vi "Logout.vi"(0 "User Manager Model in":refnum<class "User Manager Model.lvclass">, 11 "error in (no error)":errorcluster) -> (4 "User Manager Model out":refnum<class "User Manager Model.lvclass">, 15 "error out":errorcluster)   [LabVIEW 2017, in "User Manager Model.lvlib" / "User Manager Model.lvclass"]
uses:
  User Manager Model.lvclass
  C:/Program Files/National Instruments/LabVIEW 2017/vi.lib/gpm_packages/@cs/mva-core/Source/IModel/IModel/IModel.lvclass
  User Manager Model.lvclass/User Manager Model.ctl
  <vilib>/gpm_packages/@cs/persistence/source/XML/XML.lvclass
  C:/Program Files/National Instruments/LabVIEW 2017/vi.lib/gpm_packages/@cs/persistence/source/IPersist/IPersist.lvclass
  <vilib>/gpm_packages/@cs/user-manager/Source/iUser Configuration Manager/iUser Configuration Manager.lvclass
  <vilib>/gpm_packages/@cs/mva-core/Source/IObserver/IObserver/IObserver.lvclass/IObserver.ctl
  <vilib>/gpm_packages/@cs/mva-core/Source/IModel/IModel/IModel.lvclass/IModel.ctl
  <vilib>/gpm_packages/@cs/mva-core/Source/IMediator/PublishRequest/PublishRequest.lvclass/PublishRequest.ctl
  <vilib>/gpm_packages/@cs/mva-core/Source/IMediator/IMediator Messages/Publish Msg/Publish Msg.lvclass/Publish Msg.ctl
  <vilib>/gpm_packages/@cs/actor-framework-messages/Source/RoundTripMessage/RoundTripMessage.lvclass/RoundTripMessage.ctl
  <vilib>/ActorFramework/Message Enqueuer/Message Enqueuer.lvclass/Message Enqueuer.ctl
  <vilib>/gpm_packages/@cs/mva-core/Source/IMediator/IMediator Messages/Publish Msg/Send Pre-Addressed Publish.vi
  <vilib>/gpm_packages/@cs/mva-core/Source/IObserver/IObserver/Read Unique ID.vi
  <vilib>/gpm_packages/@cs/mva-core/Source/IMediator/PublishRequest/Pack Publish Request.vi
  <vilib>/gpm_packages/@cs/actor-framework-messages/Source/RoundTripMessage/Return Round-Trip Message.vi
  <vilib>/ActorFramework/Message Enqueuer/Enqueue.vi
  <vilib>/gpm_packages/@cs/mva-core/Source/IModel/IModel/IModel.lvclass
  C:/Program Files/National Instruments/LabVIEW 2017/vi.lib/gpm_packages/@cs/mva-core/Source/IObserver/IObserver/IObserver.lvclass
  <vilib>/gpm_packages/@cs/mva-core/Source/IMediator/IMediator Messages/Publish Msg/Publish Msg.lvclass
  C:/Program Files/National Instruments/LabVIEW 2017/vi.lib/gpm_packages/@cs/actor-framework-messages/Source/RoundTripMessage/RoundTripMessage.lvclass
  <vilib>/gpm_packages/@cs/actor-framework-messages/Source/RoundTripMessage/RoundTripMessage.lvclass
  C:/Program Files/National Instruments/LabVIEW 2017/vi.lib/ActorFramework/Message/Message.lvclass
  <vilib>/Utility/error.llb/Error Cluster From Error Code.vi
  <vilib>/ActorFramework/Message Priority Queue/Priority Enqueue.vi
  <vilib>/gpm_packages/@cs/mva-core/Source/IMediator/PublishRequest/PublishRequest.lvclass
  <vilib>/gpm_packages/@cs/user-manager/Source/User Configuration Manager Ref/By Ref.lvlib
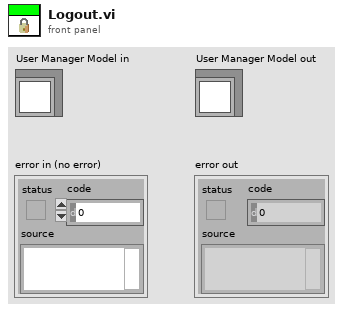
[diagram p1: front panel]
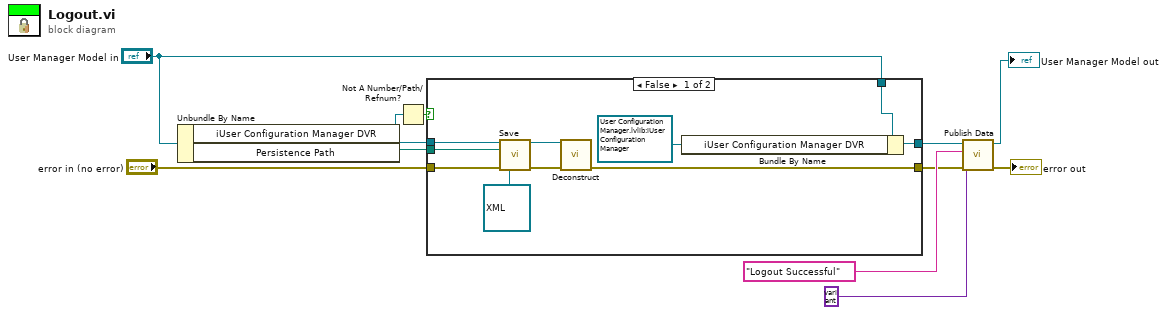
[diagram p0: block diagram]
diagram:
  n1 = Unbundle By Name("User Manager Model in") -> ("iUser Configuration Manager DVR"=w10:refnum<data-value>, "Persistence Path"=w9:path)
  n2 = Not A Number/Path/Refnum?(number/path/refnum=w10) -> (NaN/Path/Refnum?=w11:bool)
  n3 = case shown="False" w11 {
    tunnel: w10 -> [w21 _]
    tunnel: w9 -> [w20 _]
    tunnel: "error in (no error)" -> [w19 w23]
    tunnel: [w15 w23] -> w6
    tunnel: "User Manager Model in" -> [w14 w22]
    tunnel: [w12 w22] -> w3
    frame False {
      n4 = call <vilib>:"Save.vi"("iUser Configuration Manager DVR"=w21, "Path"=w20, "error in"=w19, "Persistence"=refnum<class "XML.lvclass"> refnum ("XML.lvlib:XML.lvclass")) -> ("dup iUser Configuration Manager DVR"=w17:refnum<data-value>, "error out"=w16:errorcluster)  [unwired: 10 in]
      n5 = call <vilib>:"Deconstruct.vi"("iUser Configuration Manager DVR"=w17, "Error In"=w16) -> ("Error Out"=w15:errorcluster)  [unwired: 13 in]
      n6 = Bundle By Name(cluster=w14, "iUser Configuration Manager DVR"=refnum<data-value> refnum ("dup iUser Configuration Manager DVR")) -> (w12:refnum<class "User Manager Model.lvclass">)
    }
    frame True {
    }
  }
  n7 = call <vilib>:"Publish Data.vi"("error in (no error)"=w6, "Data to Publish"=variant, "Datum Name"="Logout Successful", "IModel in"=w3) -> ("error out"=→"error out":errorcluster, "IModel out"=→"User Manager Model out":refnum<class "User Manager Model.lvclass">)  [unwired: 6 in]
